vi "SVM_Crossvalidation_FromFile.vi"(8 "error in (no error)":errorcluster) -> (0 "error out":errorcluster, 3 "Predicted labels":dbl[](array[numeric]))   [LabVIEW 2014]
uses:
  Controls/Kernel.ctl
  Wrapper API/Controls/svm_kernel_type.ctl
  Controls/Options Training.ctl
  Controls/Parameters C_SVC.ctl
  SubVIs/SVM Cross-Validate C_SVC.vi
  <userlib>/_OpenG.lib/error/error.llb/Filter Error Codes (Array)__ogtk.vi
  Tools/SubVIs/Sparse - Scale Problem Linear.vi
  Wrapper API/svm_cross_validation.vi
panel:
  in  "Param":T1={"C"=1.0, "weight_label"=[], "weight"=[]}
  in  "Nr Fold":i32=5 caption="Nr fold (LOO)"
  in  "Options":T2={"cache_size"=500.0, "eps"=0.001, "shrinking"=TRUE, "probability"=FALSE}
  in  "Kernel":T3
  out "Logging output":string
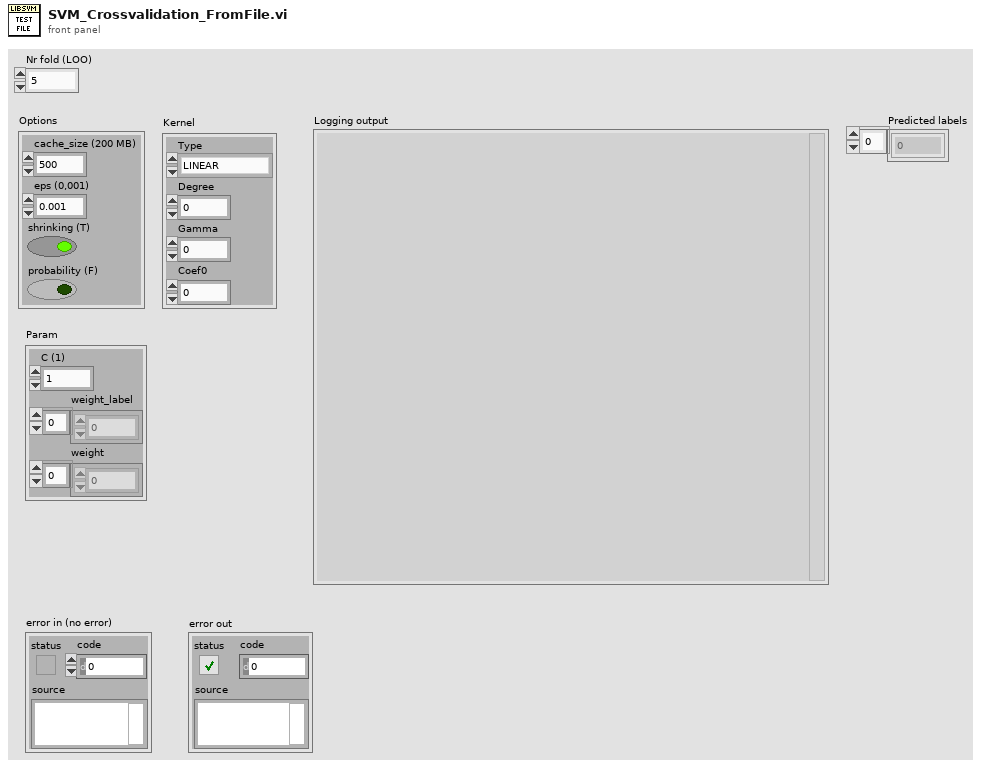
[diagram p1: front panel]
types:
  T1 = typedef "Parameters C_SVC.ctl" = cluster{"C":dbl, "weight_label":i32[], "weight":dbl[]}
  T2 = typedef "Options Training.ctl" = cluster{"cache_size":dbl, "eps":dbl, "shrinking":bool, "probability":bool}
  T3 = typedef "Kernel.ctl" = cluster{"Type":T4, "Degree":i32, "Gamma":dbl, "Coef0":dbl}
  T4 = typedef "svm_kernel_type.ctl" = enum32{"LINEAR", "POLY", "RBF", "SIGMOID", "PRECOMPUTED"}
  T5 = typedef "Logging_MessageQueue.ctl" = cluster{"Time":timestamp, "message":string}
  T6 = typedef "svm_problem.ctl" = cluster{"y":dbl[], "x":cluster{T7[]}[]}
  T7 = typedef "svm_node.ctl" = cluster{"index":i32, "value":dbl}
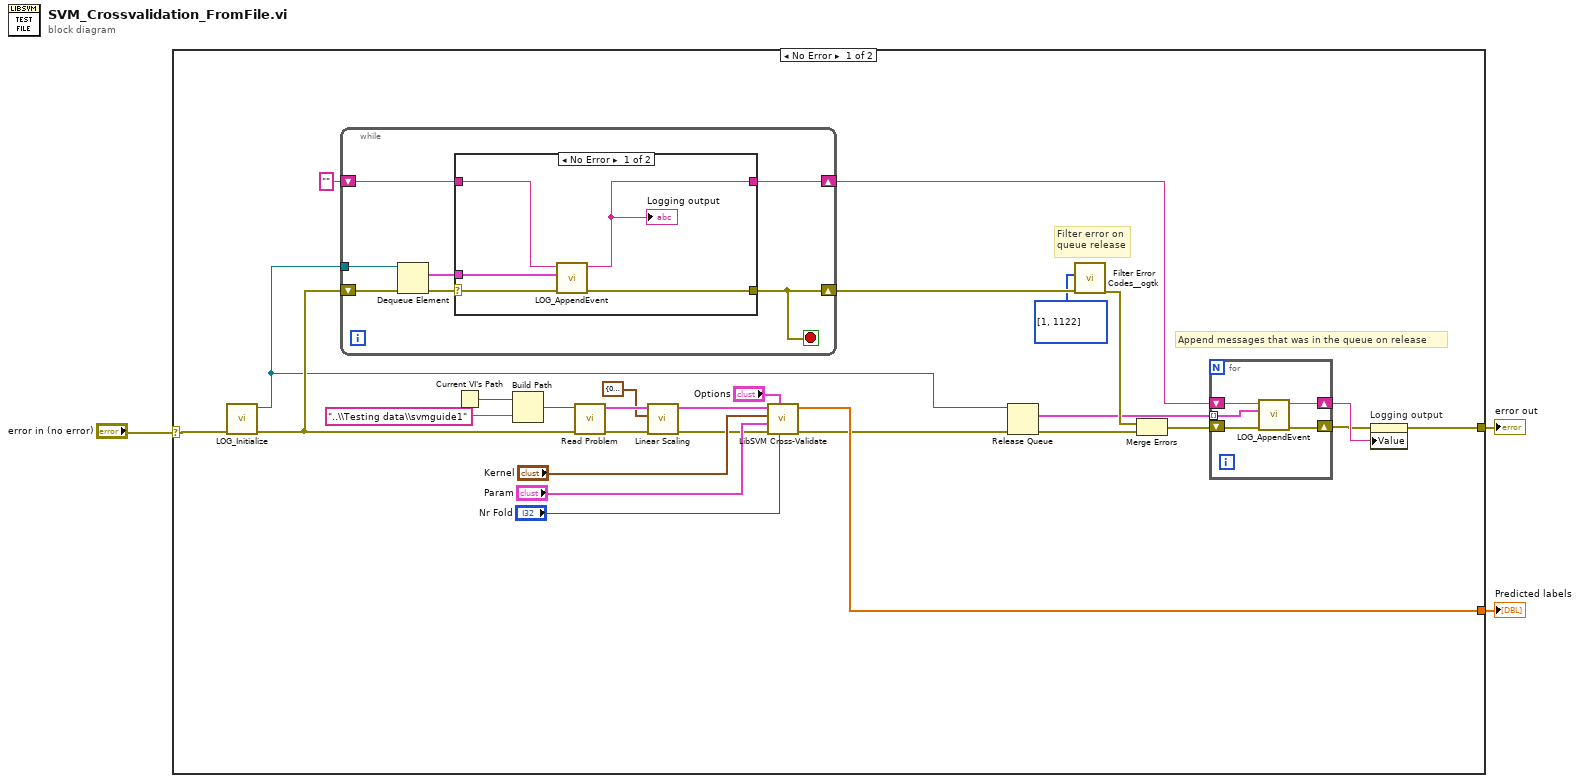
[diagram p0: block diagram]
diagram:
  n1 = case shown="No Error" "error in (no error)" {
    selector: "error in (no error)" -> [w29 w51]
    tunnel: [w17 w51] -> w1
    tunnel: [w16 _] -> w2
    frame No Error {
      # "Append messages that was in the queue on release"
      # "Filter error on\nqueue release"
      n2 = call "LOG_Initialize.vi"("error in (no error)"=w29) -> ("error out"=w27:errorcluster, "Message queue out"=w11:refnum<queue>)  [unwired: 9 in]
      n3 = while {
        tunnel: w11 -> [w43]
        shift-right: [w40] -> w20
        shift-left: "" -> [w39]
        shift-right: [w37] -> w25
        shift-left: w27 -> [w41]
        stop <- w37 stop-if-true
        n4 = Dequeue Element(queue=w43, error in (no error)=w41) -> (element=w42:T5, error out=w38:errorcluster)  [unwired: 1 in, 2 out]
        n5 = case shown="No Error" w38 {
          selector: w38 -> [w45 w50]
          tunnel: w42 -> [w48 _]
          tunnel: [w47 w49] -> w40
          tunnel: w39 -> [w46 w49]
          tunnel: [w44 w50] -> w37
          frame No Error {
            n6 = call "LOG_AppendEvent.vi"("error in (no error)"=w45, "Log Event"=w48, "String in"=w46) -> ("error out"=w44:errorcluster, "String out"=w47:string)  [unwired: 7 in]
            "Logging output" <- w47
          }
          frame Error {
          }
        }
      }
      n7 = Current VI's Path() -> (path=w30:path)
      n8 = Build Path(base path=w30, name or relative path="..\\Testing data\\svmguide1") -> (appended path=w31:path)
      n9 = call "Read Problem.vi"("error in (no error)"=w27, "file path (use dialog)"=w31) -> ("error out"=w6:errorcluster, "svm_problem"=w8:T6)  [unwired: 8 in]
      n10 = call-poly "Linear Scaling.vi"("error in (no error)"=w6, "X Scaling limits"=cluster{"X lower":dbl, "X upper":dbl} {"X lower"=0.0, "X upper"=1.0}, "Problem"=w8) -> ("error out"=w5:errorcluster, "Scaled problem"=w4:T6)  [unwired: 5 in, 2 out]
      n11 = call-poly "LibSVM Cross-Validate.vi"("Nr fold"="Nr Fold", "Options"="Options", "error in (no error)"=w5, "Param C_SVC"="Param", "Kernel"="Kernel", "Problem"=w4) -> ("error out"=w12:errorcluster, "Target"=w16:dbl[])  [unwired: 4 in]
      n12 = Release Queue(queue=w11, error in (no error)=w12) -> (remaining elements=w22:T5[], error out=w26:errorcluster)  [unwired: 1 in, 1 out]
      n13 = call-poly <userlib>:"Filter Error Codes__ogtk.vi"("Error In"=w25, "Error Codes to Filter"=i32[] [1, 1122]) -> ("Error Out"=w24:errorcluster)  [unwired: 7 in, 2 out]
      n14 = Merge Errors(w24, w26) -> (w21:errorcluster)
      n15 = for {
        tunnel: w22 -> [w35] mode=indexing
        shift-right: [w33] -> w18
        shift-left: w21 -> [w36]
        shift-right: [w32] -> w19
        shift-left: w20 -> [w34]
        n16 = call "LOG_AppendEvent.vi"("error in (no error)"=w36, "Log Event"=w35, "String in"=w34) -> ("error out"=w33:errorcluster, "String out"=w32:string)  [unwired: 7 in]
      }
      n17 = property on="Logging output" class="Str"(error in=w18, "Value"=w19) -> (error out=w17:errorcluster)  [unwired: 1 in, 1 out]
    }
    frame Error {
    }
  }
  "Predicted labels" <- w2
  "error out" <- w1
